vi "translate_inclination_to_servo_angle.vi"(2 "angle increment (0,1)":dbl=0.1 format="%#_13g", 3 "angle multiplier (4)":dbl=4.0, 4 "faster increment threshold (50)":dbl=50.0 format="%#_13g", 5 "input value":dbl format="%#_13g", 6 "input active?":bool=TRUE) -> (0 "Increment angle by":dbl)   [LabVIEW 2015]
doc: "Ouputs how much the servo angle shall be incremented/decremented based on the input value given. User may tweak the precise operation by modifying the recommended intputs.\nIf the input value is greater or equal to \"faster increment threshold\" then the angle is incremented \"angle multiplier\" times faster."
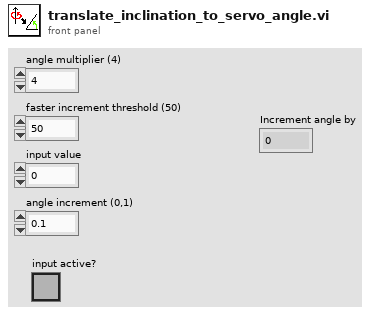
[diagram p1: front panel]
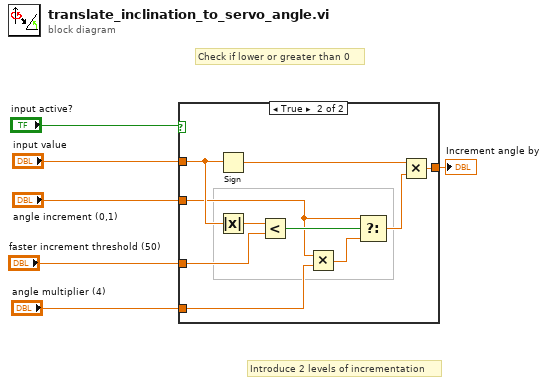
[diagram p0: block diagram]
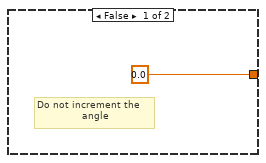
[diagram p2: hidden frame]
diagram:
  # "Introduce 2 levels of incrementation"
  # "Check if lower or greater than 0"
  n1 = case shown="True" "input active?" {
    tunnel: "input value" -> [_ w15]
    tunnel: [0.0 w16] -> w4
    tunnel: "angle increment (0,1)" -> [_ w10]
    tunnel: "faster increment threshold (50)" -> [_ w13]
    tunnel: "angle multiplier (4)" -> [_ w9]
    frame False {
      # "Do not increment the \n               angle"
    }
    frame True {
      n2 = Sign(1:w15) -> (0:w17:dbl)
      n3 = Absolute Value(x=w15) -> (abs(x)=w14:dbl)
      n4 = Less?(x=w14, y=w13) -> (x < y?=w12:bool)
      n5 = Multiply(x=w10, y=w9) -> (x*y=w8:dbl)
      n6 = Select(t=w10, s=w12, f=w8) -> (s? t:f=w11:dbl)
      n7 = Multiply(x=w17, y=w11) -> (x*y=w16:dbl)
    }
  }
  "Increment angle by" <- w4
